vi "ASIC read THx.vi"(7 "Espera acceso USB":u32=10, 8 "error in":errorcluster, 10 "Sumador":u8, 11 "ftHandle_in":u32) -> (0 "error out 2":errorcluster, 1 "THx+3":u16 format="%010b", 2 "THx":u16 format="%010b", 3 "ftHandle_out 2":u32)   [LabVIEW 2019]
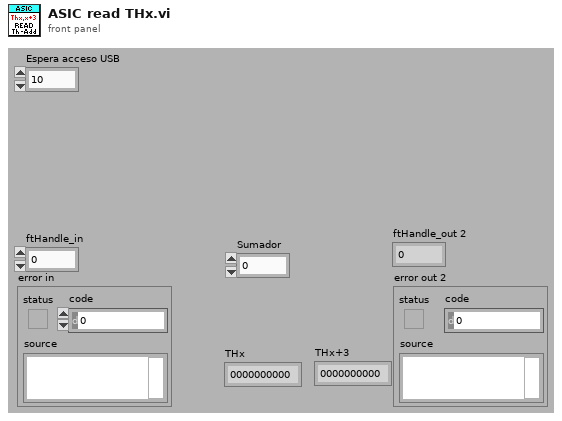
[diagram p1: front panel]
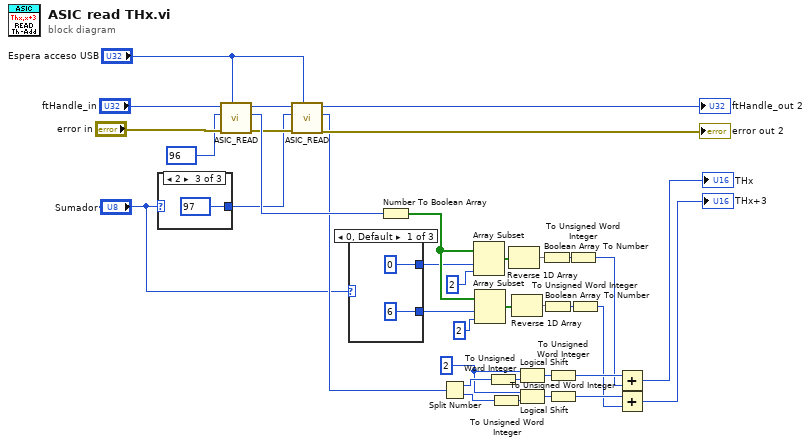
[diagram p0: block diagram]
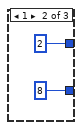
[diagram p2: hidden frame]
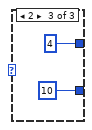
[diagram p3: hidden frame]
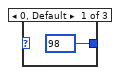
[diagram p4: hidden frame]
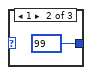
[diagram p5: hidden frame]
diagram:
  w10 = i8 2 ("y")
  n1 = case shown="2" "Sumador" {
    tunnel: [u8 98 ("Direccion Registro Asic") u8 99 ("Direccion Registro Asic") u8 97 ("Direccion Registro Asic")] -> w14
    frame 0, Default {
    }
    frame 1 {
    }
    frame 2 {
    }
  }
  n2 = call "ASIC_READ.vi"("Espera acceso USB"="Espera acceso USB", "error in"="error in", "Direccion Registro Asic"=u8 96, "ftHandle_in"="ftHandle_in") -> ("error out"=w16:errorcluster, "Valor Asic"=w18:u16, "ftHandle_out"=w17:u32)  [unwired: 5 in]
  n3 = call "ASIC_READ.vi"("Espera acceso USB"="Espera acceso USB", "error in"=w16, "Direccion Registro Asic"=w14, "ftHandle_in"=w17) -> ("error out"=→"error out 2":errorcluster, "Valor Asic"=w11:u16, "ftHandle_out"=→"ftHandle_out 2":u32)  [unwired: 5 in]
  n4 = case shown="0, Default" "Sumador" {
    tunnel: [0 ("index") 2 ("index") 4 ("index")] -> w9
    tunnel: [6 ("index") 8 ("index") 10 ("index")] -> w8
    frame 0, Default {
    }
    frame 1 {
    }
    frame 2 {
    }
  }
  n5 = Number To Boolean Array(number=w18) -> (Boolean array=w34:bool[])
  n6 = Split Number(x=w11) -> (hi(x)=w22:u8, lo(x)=w23:u8)
  n7 = Array Subset(array=w34, index=w9, length=2) -> (w4:bool[])
  n8 = Array Subset(array=w34, index=w8, length=2) -> (w2:bool[])
  n9 = To Unsigned Word Integer(number=w22) -> (unsigned 16bit integer=w36:u16)
  n10 = To Unsigned Word Integer(number=w23) -> (unsigned 16bit integer=w35:u16)
  n11 = Reverse 1D Array(array=w4) -> (reversed array=w3:bool[])
  n12 = Reverse 1D Array(array=w2) -> (reversed array=w1:bool[])
  n13 = Logical Shift(y=w10, x=w36) -> (x << y=w28:u16)
  n14 = Logical Shift(y=w10, x=w35) -> (x << y=w29:u16)
  n15 = Boolean Array To Number(Boolean array=w3) -> (number=w25:u32)
  n16 = Boolean Array To Number(Boolean array=w1) -> (number=w27:u32)
  n17 = To Unsigned Word Integer(number=w28) -> (unsigned 16bit integer=w30:u16)
  n18 = To Unsigned Word Integer(number=w29) -> (unsigned 16bit integer=w31:u16)
  n19 = To Unsigned Word Integer(number=w25) -> (unsigned 16bit integer=w5:u16)
  n20 = To Unsigned Word Integer(number=w27) -> (unsigned 16bit integer=w6:u16)
  n21 = Add(x=w30, y=w5) -> (x+y=→"THx":u16)
  n22 = Add(x=w31, y=w6) -> (x+y=→"THx+3":u16)
